vi "Get Error Queue Name.vi"(7 "Action":enum16{"Get", "Set"}(ring), 8 "error in (no error)":errorcluster, 11 "Queue Name":string) -> (0 "error out":errorcluster, 3 "Queue Name":string)   [LabVIEW 2020, in "Error Handler.lvclass"]
uses:
  Error Handler.lvclass
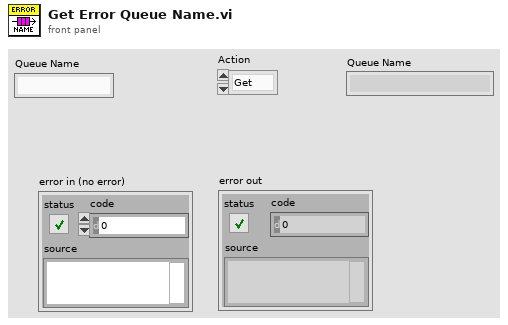
[diagram p1: front panel]
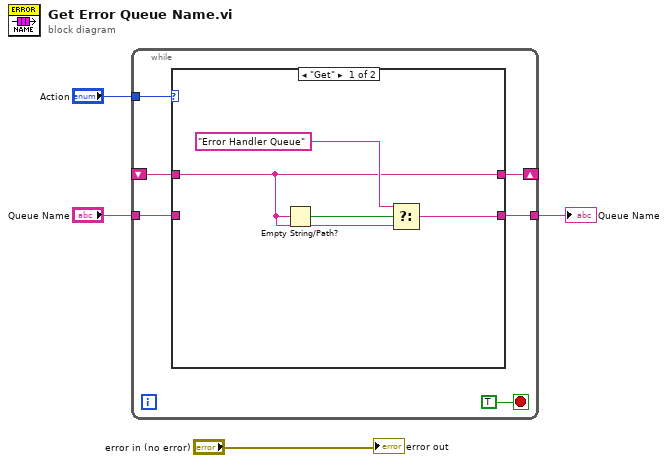
[diagram p0: block diagram]
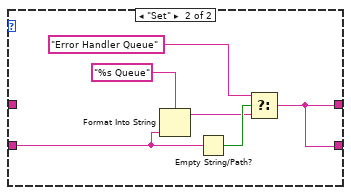
[diagram p2: hidden frame]
diagram:
  n1 = while {
    shift-right: [w10] -> _
    shift-left: _ -> [w7]
    tunnel: "Action" -> [w8]
    tunnel: "Queue Name" -> [w6]
    tunnel: [w5] -> w2
    stop <- TRUE stop-if-true
    n2 = case shown="\"Get\"" w8 {
      tunnel: [w12 w15] -> w10
      tunnel: w7 -> [w12 _]
      tunnel: w6 -> [_ w19]
      tunnel: [w11 w15] -> w5
      frame "Get" {
        n3 = Empty String/Path?(string/path=w12) -> (empty?=w14:bool)
        n4 = Select(t="Error Handler Queue", s=w14, f=w12) -> (s? t:f=w11:string)
      }
      frame "Set" {
        n5 = Format Into String(format string="%s Queue", w19) -> (resulting string=w17:string)  [unwired: 2 in, 1 out]
        n6 = Empty String/Path?(string/path=w19) -> (empty?=w18:bool)
        n7 = Select(t="Error Handler Queue", s=w18, f=w17) -> (s? t:f=w15:string)
      }
    }
  }
  "Queue Name" <- w2
  "error out" <- "error in (no error)"
